vi "PH_SHS_Analysis_Statistician.constructor.vi"(0 "name":string, 2 "data in":string, 5 "error in":errorcluster) -> (14 "i ref out":refnum<vi>, 16 "data out":string, 19 "error out":errorcluster)   [LabVIEW 2014, in "PH_SHS_Analysis_Statistician.lvlib"]
doc: "author: Stefan Götte, GSI\n\nLicense Agreement for this software:\n\nCopyright (C)\nGesellschaft für Schwerionenforschung, GSI\nPlanckstr. 1\n64291 Darmstadt\nGermany\n\nContact: D.Beck@gsi.de \n\nThis program is free software; you can redistribute it and/or modify it under the terms of the \nGNU General Public License as published by the Free Software Foundation; either version 2 of \nthe license, or (at your option) any later version.\n\nThis program is distributed in the hope that it will be useful, but WITHOUT ANY WARRANTY; \nwithout even the implied warranty of MERCHANTABILITY or FITNESS FOR A PARTICULAR PURPOSE. See the GNU General License for more details (http://www.gnu.org).\n\nGesellschaft für Schwerionenforschung, GSI\nPlanckstr. 1, 64291 Darmstadt, Germany\nFor all questions and ideas contact: M.Richter@gsi.de, H.Brand@gsi.de or D.Beck@gsi.de.\nLast update: 16-JUN-2004"
uses:
  PH_SHS_Analysis_Statistician.lvlib
  CSCore/CSObj/CSObj.lvlib
  PH_Class/PH_Class.lvlib
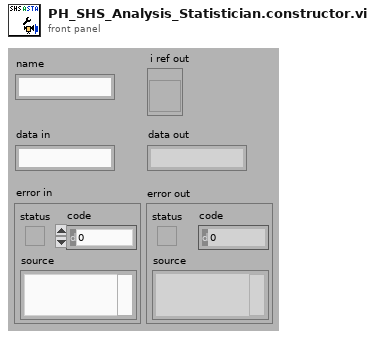
[diagram p1: front panel]
types:
  T1 = enum16{"SetAttribute", "GetAttribute", "CreateAttribute", "DestroyAttribute", "DestroyAllAtributes"}
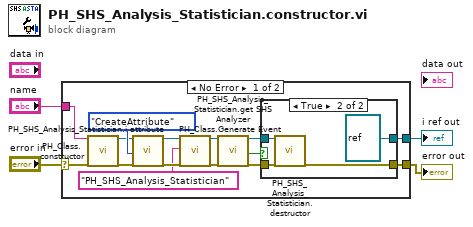
[diagram p0: block diagram]
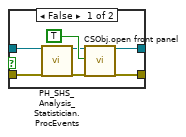
[diagram p2: hidden frame]
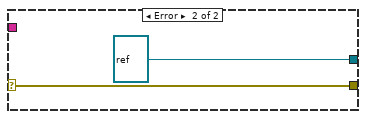
[diagram p3: hidden frame]
diagram:
  n1 = case shown="No Error" "error in" {
    selector: "error in" -> [w13 w32]
    tunnel: "name" -> [w9 _]
    tunnel: [w8 refnum<vi> refnum ("i ref out")] -> w3
    tunnel: [w7 w32] -> w2
    frame No Error {
      n2 = call "PH_Class.constructor.vi"("name"=w9, "error in"=w13) -> ("i ref out"=w18:refnum<vi>, "error out"=w17:errorcluster)  [unwired: 15 in, 1 out]
      n3 = call "PH_SHS_Analysis_Statistician.i attribute.vi"("VI Refnum"=w18, "Action"=T1."CreateAttribute", "error in (no error)"=w17) -> ("VI Refnum out"=w16:refnum<vi>, "error out"=w6:errorcluster)  [unwired: 14 in, 1 out]
      n4 = call "PH_Class.Generate Event.vi"("i ref in"=w16, "Class"="PH_SHS_Analysis_Statistician", "error in (no error)"=w6) -> ("i ref out"=w15:refnum<vi>, "error out"=w14:errorcluster)  [unwired: 15 in]
      n5 = call "PH_SHS_Analysis_Statistician.get SHS Analyzer.vi"("i ref in"=w15, "error in"=w14) -> ("i ref out"=w11:refnum<vi>, "No Analyzer selected?"=w10:bool, "error out"=w12:errorcluster)  [unwired: 15 in]
      n6 = case shown="True" w10 {
        tunnel: [w26 w28] -> w7
        tunnel: [w25 refnum<vi> refnum ("i ref out")] -> w8
        tunnel: w12 -> [w23 w29]
        tunnel: w11 -> [w21 w30]
        frame False {
          n7 = call "PH_SHS_Analysis_Statistician.ProcEvents.vi"("i ref in"=w21, "error in (no error)"=w23) -> ("i ref out"=w20:refnum<vi>, "error out"=w22:errorcluster)  [unwired: 16 in]
          n8 = call "CSObj.open front panel.vi"("i ref in"=w20, "frontPanelOpen"=TRUE ("front panel open"), "error in (no error)"=w22) -> ("i ref out"=w25:refnum<vi>, "error out"=w26:errorcluster)  [unwired: 15 in]
        }
        frame True {
          n9 = call "PH_SHS_Analysis_Statistician.destructor.vi"("i ref in"=w30, "error in(no error)"=w29) -> ("error out"=w28:errorcluster)  [unwired: 17 in]
        }
      }
    }
    frame Error {
    }
  }
  "i ref out" <- w3
  "error out" <- w2
